vi "Initialize HDF5 file.vi"(8 "error in (no error)":errorcluster, 10 "Save data? in":bool, 11 "Save data path in":path) -> (0 "error out":errorcluster, 1 "HDF5 Dataset Ref out":T1, 2 "Save data? out":bool, 3 "HDF5 Ref out":T1)   [LabVIEW 2018]
uses:
  <vilib>/UPVI/lvhdf5/library.llb/HDF5 Ref.ctl
  <vilib>/UPVI/lvhdf5/file.llb/LVH5F Operation.ctl
  <vilib>/UPVI/lvhdf5/dataset.llb/LVH5D Operation.ctl
  <vilib>/UPVI/lvhdf5/dataset.llb/Simple OpenCreateReplace Dataset (Variant).vi
  <vilib>/UPVI/lvhdf5/dataset.llb/Simple OpenCreateReplace Dataset.xnode
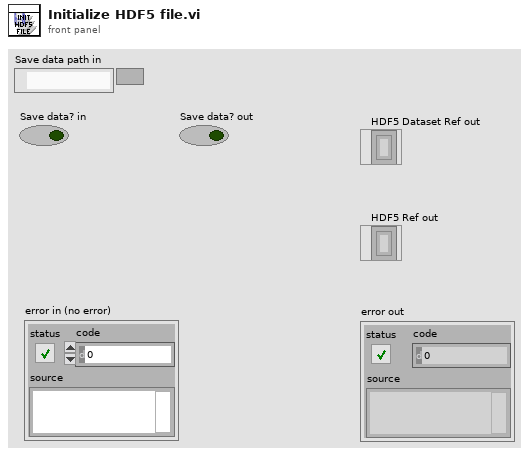
[diagram p1: front panel]
types:
  T1 = typedef "HDF5 Ref.ctl" = refnum<k1>
  T2 = typedef "LVH5D Operation.ctl" = enum16{"open", "replace", "create", "open or create", "create or replace", "create or replace with confirmation"}
  T3 = typedef "LVH5F Operation.ctl" = enum16{"open", "open or create", "create or replace", "create or replace (with confirmation)", "create", "open (read only)"}
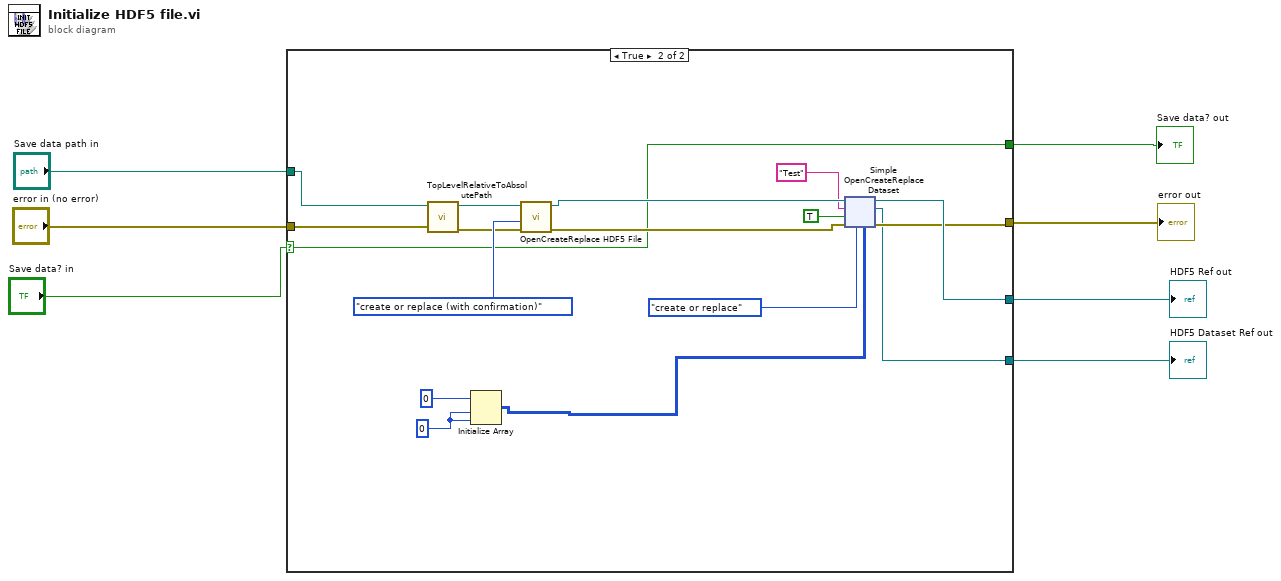
[diagram p0: block diagram]
diagram:
  n1 = case shown="True" "Save data? in" {
    selector: "Save data? in" -> [w9 w17]
    tunnel: "Save data path in" -> [_ w24]
    tunnel: [w9 w17] -> w5
    tunnel: [w8 w15] -> w4
    tunnel: "error in (no error)" -> [w8 w23]
    tunnel: [_ w16] -> w2
    tunnel: [_ w14] -> w1
    frame False {
    }
    frame True {
      w10 = 0 ("dimension size")
      n2 = call "TopLevelRelativeToAbsolutePath.vi"("error in (no error)"=w23, "Path Relative to Top Level VI"=w24) -> ("error out"=w22:errorcluster, "Absolute path"=w25:path)  [unwired: 8 in]
      n3 = Initialize Array(i16 0, w10, w10) -> (w11:i16[][])
      n4 = call <vilib>:"OpenCreateReplace HDF5 File.vi"("error in (no error)"=w22, "function (open or create)"=LVH5F_Operation."create or replace (with confirmation)", "path"=w25) -> ("error out"=w19:errorcluster, "HDF5 Ref out"=w20:T1)  [unwired: 5 in]
      n5 = xnode "Simple OpenCreateReplace Dataset"("Dataset Path"="Test", "HDF5 Ref"=w20, "Unlimited  dataset (F)"=TRUE, "error in (no error)"=w19, "operation"=LVH5D_Operation."create or replace", "Datatype and Dataspace"=w11) -> ("HDF5 Dataset Ref out"=w14:T1, "HDF5 Ref out"=w16:T1, "error out"=w15:errorcluster)  [unwired: 2 in]
    }
  }
  "Save data? out" <- w5
  "error out" <- w4
  "HDF5 Ref out" <- w2
  "HDF5 Dataset Ref out" <- w1
